vi "SeqMgr.If Statement, Find End after Else.vi"(9 "Arguements":string[](array[string]), 10 "Next Step":i32, 11 "Sequence":string[][](array[string])) -> (0 "error out":errorcluster, 2 "Next Step":i32, 3 "End":bool)   [LabVIEW 2024, in "EQMF.lvlib" / "SeqMgr.lvlib"]
uses:
  SeqMgr.lvlib
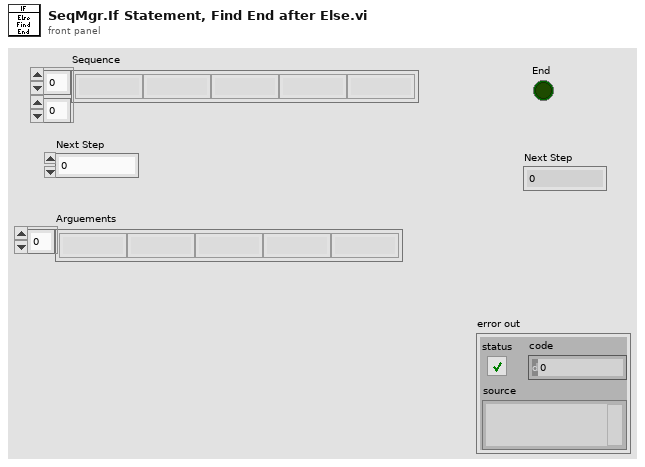
[diagram p1: front panel]
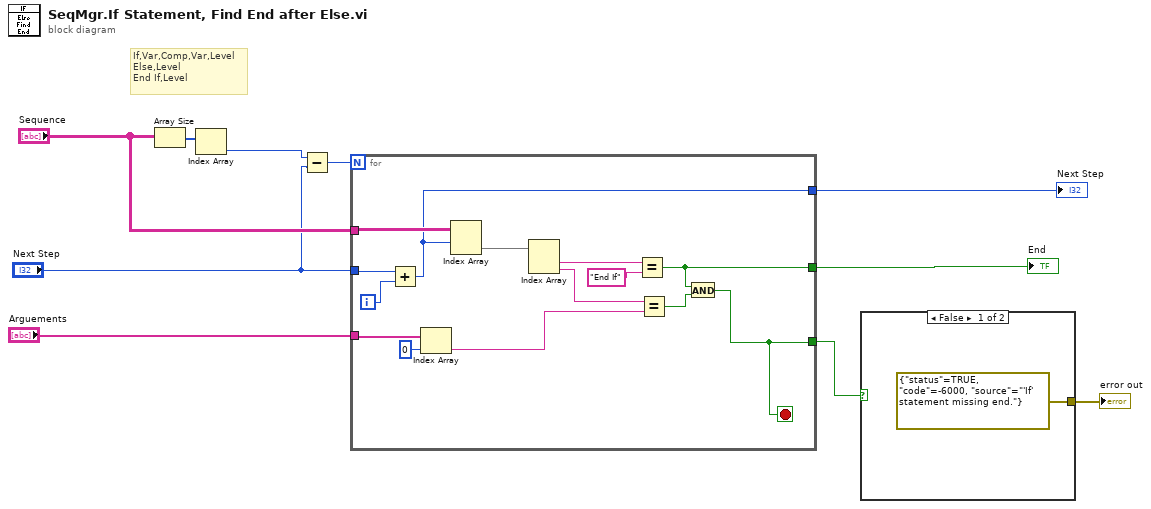
[diagram p0: block diagram]
diagram:
  # "If,Var,Comp,Var,Level\nElse,Level\nEnd If,Level"
  n1 = Array Size(array="Sequence") -> (size(s)=w6:i32[])
  n2 = Index Array(array=w6) -> (element=w1:i32)  [unwired: 1 in]
  n3 = Subtract(x=w1, y="Next Step") -> (x-y=w5:i32)
  n4 = for {
    N: w5 -> [_]
    tunnel: "Next Step" -> [w24]
    tunnel: "Sequence" -> [w22]
    tunnel: "Arguements" -> [w19]
    tunnel: [w14] -> w8
    tunnel: [w11] -> w2
    tunnel: [w12] -> w3
    i -> [w23]
    stop <- w11 stop-if-true
    n5 = Add(x=w24, y=w23) -> (x+y=w14:i32)
    n6 = Index Array(array=w19, index=0) -> (element=w15:string)
    n7 = Index Array(array=w22, index (row)=w14) -> (element=w21:string[])  [unwired: 1 in]
    n8 = Index Array(array=w21) -> (element #1=w13:string, element #2=w16:string)  [unwired: 2 in]
    n9 = Equal?(x=w13, y="End If") -> (x = y?=w12:bool)
    n10 = Equal?(x=w16, y=w15) -> (x = y?=w17:bool)
    n11 = And(x=w12, y=w17) -> (x .and. y?=w11:bool)
  }
  "End" <- w3
  "Next Step" <- w8
  n12 = case shown="False" w2 {
    tunnel: [errorcluster {"status"=TRUE, "code"=-6000, "source"="'If' statement missing end."} ("error constant") _] -> w4
    frame False {
    }
    frame True {
    }
  }
  "error out" <- w4
